vi "GetMLP.vi"(10 "Particle Reports (Pixels)":T2(array[cluster]) {"Orientation" format="%.2f"; "Dimensions"."Height" format="%.2f"; "Dimensions"."Width" format="%.2f"; "Center of Mass"."Y" format="%.2f"; "Center of Mass"."X" format="%.2f"; "Bounding Rect"."Bottom" format="%.2f"; "Bounding Rect"."Right" format="%.2f"; "Bounding Rect"."Top" format="%.2f"; "Bounding Rect"."Left" format="%.2f"; "Number of Holes" format="%.2f"; "Area" format="%.2f"}) -> (2 "MLP Report":T1 {"Orientation" format="%.2f"; "Dimensions"."Height" format="%.2f"; "Dimensions"."Width" format="%.2f"; "Center of Mass"."Y" format="%.2f"; "Center of Mass"."X" format="%.2f"; "Bounding Rect"."Bottom" format="%.2f"; "Bounding Rect"."Right" format="%.2f"; "Bounding Rect"."Top" format="%.2f"; "Bounding Rect"."Left" format="%.2f"; "Number of Holes" format="%.2f"; "Area" format="%.2f"})   [LabVIEW 2014]
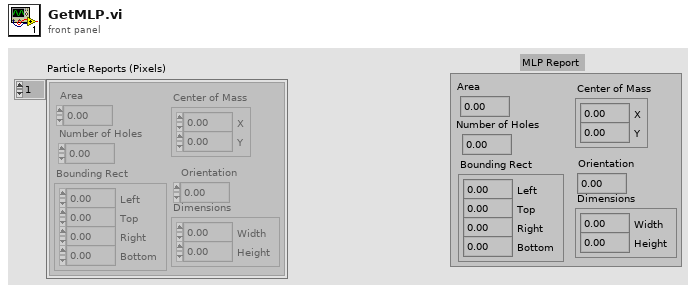
[diagram p1: front panel]
types:
  T1 = cluster{"Area":dbl, "Number of Holes":dbl, "Bounding Rect":cluster{"Left":dbl, "Top":dbl, "Right":dbl, "Bottom":dbl}, "Center of Mass":cluster{"X":dbl, "Y":dbl}, "Orientation":dbl, "Dimensions":cluster{"Width":dbl, "Height":dbl}}
  T2 = cluster{"Area":dbl, "Number of Holes":dbl, "Bounding Rect":cluster{"Left":dbl, "Top":dbl, "Right":dbl, "Bottom":dbl}, "Center of Mass":cluster{"X":dbl, "Y":dbl}, "Orientation":dbl, "Dimensions":cluster{"Width":dbl, "Height":dbl}}[]
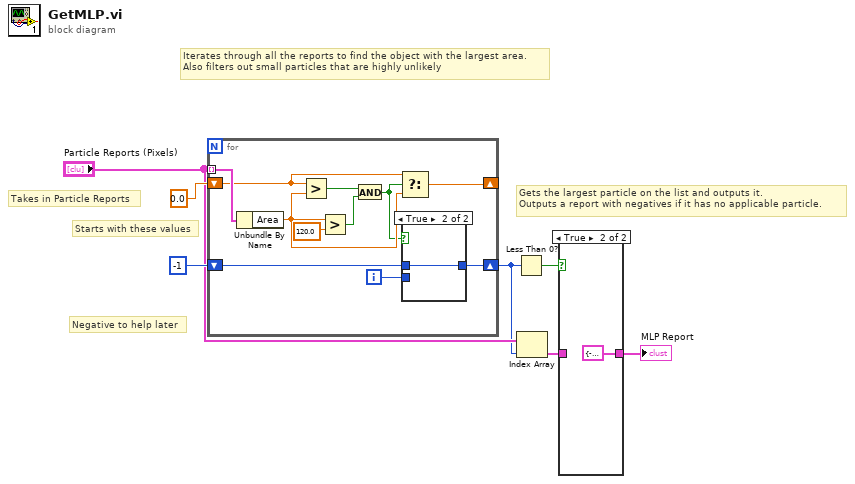
[diagram p0: block diagram]
diagram:
  # "Gets the largest particle on the list and outputs it.\nOutputs a report with negatives if it has no applicable particle."
  # "Negative to help later"
  # "Starts with these values"
  # "Iterates through all the reports to find the object with the largest area.\nAlso filters out small particles that are highly unlikely"
  # "Takes in Particle Reports"
  n1 = for {
    tunnel: "Particle Reports (Pixels)" -> [w18] mode=indexing
    shift-right: [w16] -> _
    shift-left: 0.0 -> [w17]
    shift-right: [w13] -> w4
    shift-left: -1 -> [w14]
    i -> [w15]
    n2 = Unbundle By Name(w18) -> ("Area"=w10:dbl)
    n3 = Greater?(x=w17, y=w10) -> (0:w12:bool)
    n4 = Greater?(x=w10, y=120.0) -> (0:w11:bool)
    n5 = And(x=w12, y=w11) -> (x .and. y?=w8:bool)
    n6 = Select(t=w17, s=w8, f=w10) -> (s? t:f=w16:dbl)
    n7 = case shown="True" w8 {
      tunnel: w15 -> [w19 _]
      tunnel: w14 -> [_ w20]
      tunnel: [w19 w20] -> w13
      frame False {
      }
      frame True {
      }
    }
  }
  n8 = Less Than 0?(x=w4) -> (x < 0?=w3:bool)
  n9 = Index Array(array="Particle Reports (Pixels)", index=w4) -> (element=w1:T1)
  n10 = case shown="True" w3 {
    tunnel: [w21 T1 {"Area"=-1.0, "Number of Holes"=-1.0, "Bounding Rect"={"Left"=-1.0, "Top"=-1.0, "Right"=-1.0, "Bottom"=-1.0}, "Center of Mass"={"X"=-1.0, "Y"=-1.0}, "Orientation"=-1.0, "Dimensions"={"Width"=-1.0, "Height"=-1.0}} ("MLP Report 2")] -> w2
    tunnel: w1 -> [w21 _]
    frame False {
    }
    frame True {
    }
  }
  "MLP Report" <- w2
